vi "WPI_UtilitiesStartTest.vi"(11 "String":string) -> (0 "error out":errorcluster, 3 "Name":string)   [LabVIEW 2017]
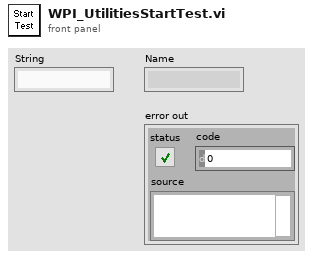
[diagram p1: front panel]
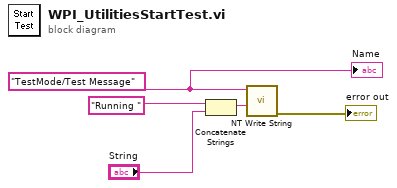
[diagram p0: block diagram]
diagram:
  w5 = "TestMode/Test Message" ("Name")
  n1 = Concatenate Strings("Running " ("Name"), "String") -> (w2:string)
  n2 = call <vilib>:"NT Write String.vi"("String"=w2, "Name"=w5) -> ("error out"=→"error out":errorcluster)  [unwired: 9 in]
  "Name" <- w5
